vi "Append Line.vi"(0 "PDF Report IN":T22(xcontrol), 1 "Line cluster":T1={"Thickness (point)"=0.75, "Alighment"=enum."Right", "%width"=100.0, "Color"=1, "X Offset (point)"=0.0, "Y Offset (point)"=-6.0} {"%width" min=0 max=100 format="%#.0f"}, 11 "error in (no error)":errorcluster) -> (4 "PDF Report OUT":T22(xcontrol), 15 "error out":errorcluster)   [LabVIEW 2013]
doc: "<B>ENGLISH</B>\nAppends a <B>horizontal line</B> to the PDF report.\n\n<B>FRANÇAIS</B>\nAjoute une <B>ligne horizontale</B> au rapport PDF.\n\nDeveloped by Jean-Marc Simard\nCopyright © 2010, Exaprom Inc.\nAll rights reserved.\nLicense: BSD\n\nWith iTextSharp 4.1.6 (http://itextsharp.sourceforge.net)\nunder Mozilla Public License Version 1.1\n(http://www.mozilla.org/MPL/MPL-1.1.html)"
uses:
  C:/Users/MaxCorp/Documents/GitHub/TopView/DLL/itextsharp.dll
  DLL/itextsharp.dll
  Controls/CB SetColor.ctl
  Controls/Line cluster.ctl
  Controls/PDF Report Xcontrol/PDF Report.xctl
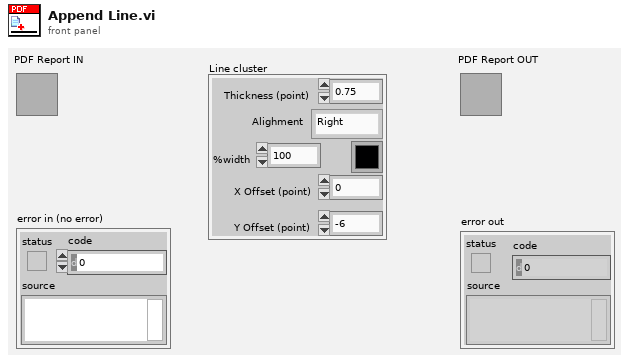
[diagram p1: front panel]
types:
  T1 = typedef "Line cluster.ctl" = cluster{"Thickness (point)":sgl, "Alighment":enum16{"Left", "Center", "Right"}, "%width":sgl, "Color":u32, "X Offset (point)":sgl, "Y Offset (point)":sgl}
  T2 = typedef "Font cluster.ctl" = cluster{"Name":string, "Size":T3, "Color":T4, "Style":cluster{"Bold":bool, "Italic":bool, "Underline":bool, "Strikeout":bool}}
  T3 = typedef "Font size.ctl" = sgl
  T4 = typedef "Font color.ctl" = u32
  T5 = typedef "Unit.ctl" = enum16{"inch", "mm"}
  T6 = typedef "Paragraphe cluster.ctl" = cluster{" Aligment":T7, "Line spacing":T8}
  T7 = typedef "Texte alignement.ctl" = enum16{"Select", "CENTER", "JUSTIFY", "LEFT", "RIGHT"}
  T8 = typedef "Line spacing.ctl" = enum16{"Select", "1.0", "1.5", "2.0"}
  T9 = typedef "Page dimensions.ctl" = cluster{"Start at page":i32, "Orientation":T10, "widht":sgl, "height":sgl, "Margin left":sgl, "Margin right":sgl, "Margin top":sgl, "Margin bottom":sgl}
  T10 = typedef "Page Orientation.ctl" = enum16{"Portrait", "Landscape"}
  T11 = typedef "Image or Table Caption.ctl" = cluster{"Caption":string, "Separator":string, "Position":enum16{"Above", "Below"}}
  T12 = typedef "Header Footer [ ].ctl" = T13[]
  T13 = typedef "Header Footer cluster.ctl" = cluster{"Start page":i32, "Type":T14, "Alignment":T15, "Vertical Alignement":T16, "Image (%)":sgl, "Page #":T17, "Text":string, "Path":string, "Font":T2, "Font refnum":refnum<k24>, "Line":cluster{"Line":T18, "Thickness (points)":sgl, "Colour":T4}}
  T14 = typedef "Header Footer Type.ctl" = enum16{"Select", "Text", "Text + hyperlink", "Page number", "Image", "Image + hyperlink"}
  T15 = typedef "Header footer horiz alignment.ctl" = enum16{"Left", "Center", "Right"}
  T16 = typedef "Cell Vertical alignment.ctl" = enum16{"TOP", "MIDDLE", "BOTTOM"}
  T17 = typedef "Page number.ctl" = cluster{"Text 1":string, "Text 2":string, "Text 3":string}
  T18 = typedef "Header Footer Line.ctl" = enum16{"No line", "Horizontal line"}
  T19 = typedef "Watermark cluster2.ctl" = cluster{"Show? (F)":bool, "Type":enum16{"Image", "Text"}, "Opacity (%)":sgl, "Rotate(°)":sgl, "Position":cluster{"Position":T20, "X":sgl, "Y":sgl}, "Image path":path, "Scaled(%)":sgl, "Image refnum":refnum<k24>, "Text":string, "Font":cluster{"Name":string, "Size":T3, "Color":T4}, "Font refnum":refnum<k24>, "Alignment":T15, "Automatic":bool}
  T20 = typedef "Watermark Position.ctl" = enum16{"Absolute", "Center (page)", "Center (text section)"}
  T21 = typedef "System Fonts.ctl" = cluster{"Font name [ ]":string[], "Font and file names [ ]":cluster{"Font name":string, "File name":string}[]}
  T22 = cluster{"Document":refnum<k24>, "Writer":refnum<k24>, "Default Font":refnum<k24>, "Default Font cluster":T2, "Path":path, "Unit (default = mm)":T5, "Paragraphe cluster":T6, "Pages dimensions [ ]":T9[], "Captions":cluster{"Image":T11, "Image counter":u16, "Table":T11, "Table counter":u16, "Font":T2}, "Header":T12, "Footer":T12, "Watermark ":T19, "Actual VI name":string, "System Fonts":T21}
  T23 = typedef "CB SetColor.ctl" = enum16{"Fill", "Stroke"}
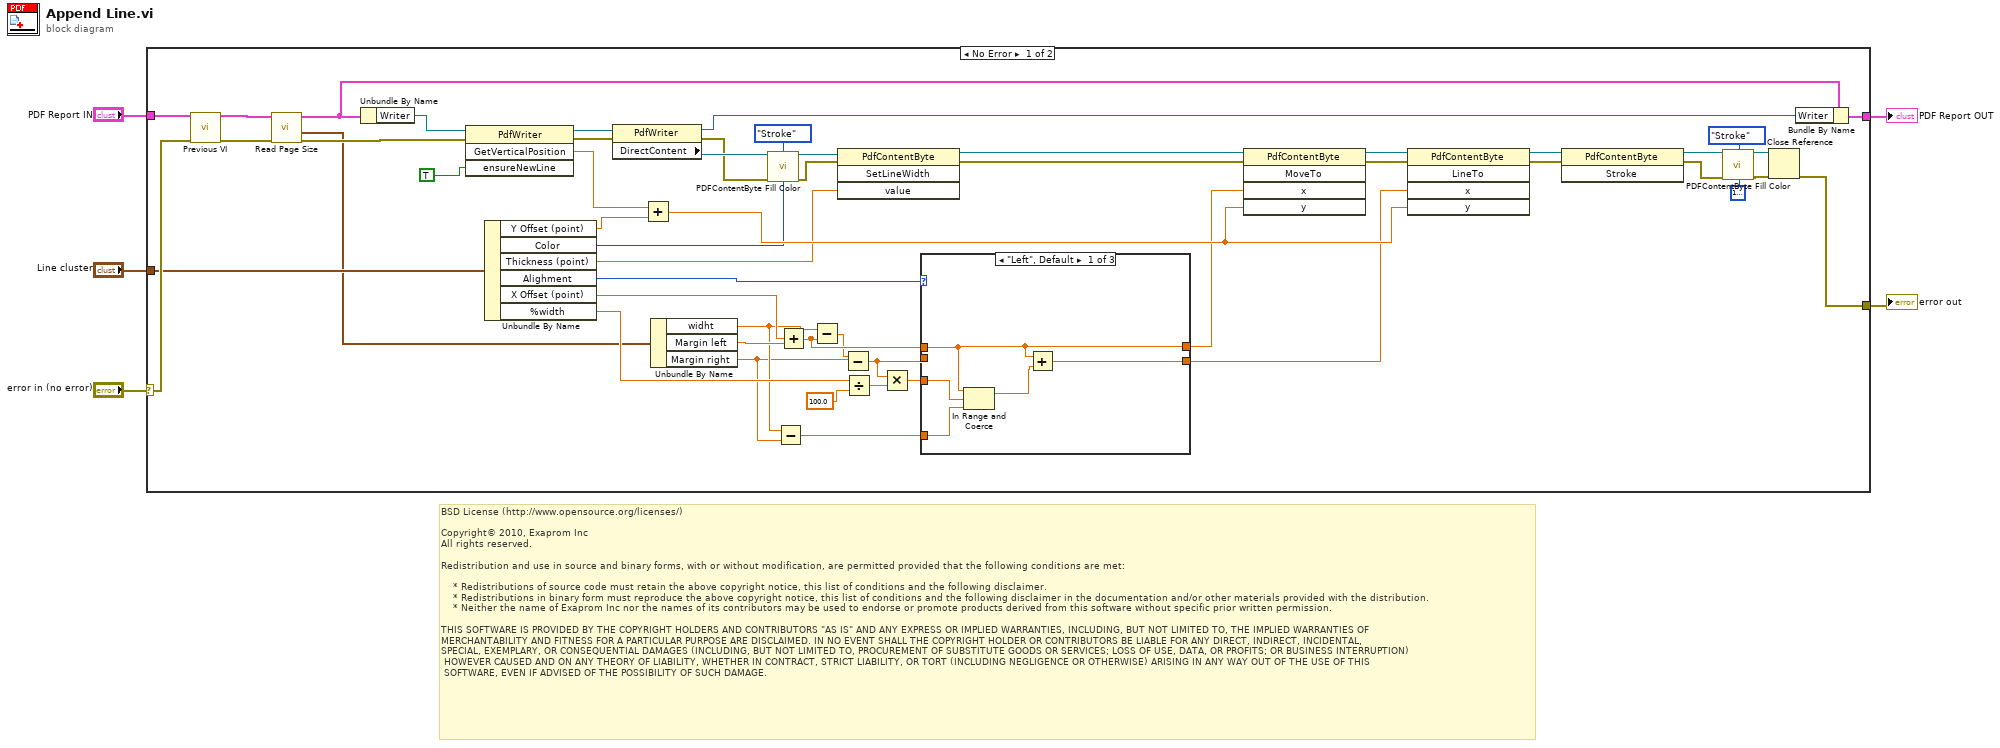
[diagram p0: block diagram]
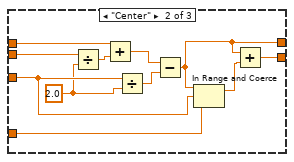
[diagram p2: hidden frame]
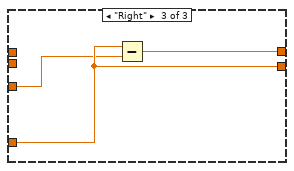
[diagram p3: hidden frame]
diagram:
  # "BSD License (http://www.opensource.org/licenses/)\n\nCopyright© 2010, Exaprom Inc\nAll rights reserved.\n\nRedistribution and use in source and binary forms, with or without modification, are permitted provided that the following conditions are met:\n\n    * Redistributions of source code must retain the above copyright notice, this list of conditions and the following disclaimer.\n    * Redistributions in binary form must reproduce the above copyright notice, this list of conditions and the following disclaimer in the documentation and/or other materials provided with the distribution.\n    * Neither the name of Exaprom Inc nor the names of its contributors may be used to endorse or promote products derived from this software without specific prior written permission.\n\nTHIS SOFTWARE IS PROVIDED BY THE COPYRIGHT HOLDERS AND CONTRIBUTORS \"AS IS\" AND ANY EXPRESS OR IMPLIED WARRANTIES, INCLUDING, BUT NOT LIMITED TO, THE IMPLIED WARRANTIES OF \nMERCHANTABILITY AND FITNESS FOR A PARTICULAR PURPOSE ARE DISCLAIMED. IN NO EVENT SHALL THE COPYRIGHT HOLDER OR CONTRIBUTORS BE LIABLE FOR ANY DIRECT, INDIRECT, INCIDENTAL,\nSPECIAL, EXEMPLARY, OR CONSEQUENTIAL DAMAGES (INCLUDING, BUT NOT LIMITED TO, PROCUREMENT OF SUBSTITUTE GOODS OR SERVICES; LOSS OF USE, DATA, OR PROFITS; OR BUSINESS INTERRUPTION)\n HOWEVER CAUSED AND ON ANY THEORY OF LIABILITY, WHETHER IN CONTRACT, STRICT LIABILITY, OR TORT (INCLUDING NEGLIGENCE OR OTHERWISE) ARISING IN ANY WAY OUT OF THE USE OF THIS\n SOFTWARE, EVEN IF ADVISED OF THE POSSIBILITY OF SUCH DAMAGE."
  n1 = case shown="No Error" "error in (no error)" {
    selector: "error in (no error)" -> [w57 w78]
    tunnel: [w20 w78] -> w5
    tunnel: "PDF Report IN" -> [w24 w77]
    tunnel: [w27 w77] -> w2
    tunnel: "Line cluster" -> [w42 _]
    frame No Error {
      n2 = call "Previous VI.vi"("PDF Report IN"=w24, "error in (no error)"=w57) -> ("PDF Report OUT"=w7:T22, "error out"=w6:errorcluster)  [unwired: 12 out]
      n3 = call "Read Page Size.vi"("error in (no error)"=w6, "PDF Report"=w7) -> ("error out"=w22:errorcluster, "Page (points)"=w21:T9, "PDF Report duplicate"=w23:T22)  [unwired: 7 out]
      n4 = Unbundle By Name(w23) -> ("Writer"=w26:refnum<k24>)
      n5 = invoke class="PdfWriter" method="GetVerticalPosition"(reference=w26, error in=w22, "ensureNewLine"=TRUE) -> (reference out=w55:refnum<k24>, error out=w56:errorcluster, "GetVerticalPosition"=w49:sgl)  [unwired: 1 in, 1 out]
      n6 = Unbundle By Name(w42) -> ("Y Offset (point)"=w41:sgl, "Color"=w10:u32, "Thickness (point)"=w40:sgl, "Alighment"=w38:enum16{"Left", "Center", "Right"}, "X Offset (point)"=w36:sgl, "%width"=w39:sgl)
      n7 = property class="PdfWriter"(reference=w55, error in=w56) -> (reference out=w25:refnum<k24>, error out=w12:errorcluster, "DirectContent"=w13:refnum<k24>)
      n8 = Add(x=w49, y=w41) -> (x+y=w48:sgl)
      n9 = Unbundle By Name(w21) -> ("widht"=w34:sgl, "Margin left"=w37:sgl, "Margin right"=w32:sgl)
      n10 = call "PDFContentByte Fill Color.vi"("PDFContentByte"=w13, "CB SetColor"=CB_SetColor."Stroke", "error in (no error)"=w12, "Color Box"=w10) -> ("PDFContentByte duplicate"=w14:refnum<k24>, "error out"=w11:errorcluster)  [unwired: 10 out]
      n11 = Subtract(x=w34, y=w32) -> (x-y=w33:sgl)
      n12 = Add(x=w36, y=w37) -> (x+y=w35:sgl)
      n13 = Subtract(x=w34, y=w35) -> (x-y=w31:sgl)
      n14 = invoke class="PdfContentByte" method="SetLineWidth"(reference=w14, error in=w11, "value"=w40) -> (reference out=w29:refnum<k24>, error out=w28:errorcluster)  [unwired: 1 in, 2 out]
      n15 = Subtract(x=w31, y=w32) -> (x-y=w30:sgl)
      n16 = Divide(x=w39, y=sgl 100.0) -> (x/y=w43:sgl)
      n17 = Multiply(x=w30, y=w43) -> (x*y=w46:sgl)
      n18 = case shown="\"Left\", Default" w38 {
        tunnel: w35 -> [w60 w69 _]
        tunnel: [w60 w66 w75] -> w47
        tunnel: w46 -> [w59 w65 w74]
        tunnel: [w62 w73 w76] -> w45
        tunnel: w33 -> [w61 w64 w76]
        tunnel: w30 -> [_ w71 _]
        frame "Left", Default {
          n19 = In Range and Coerce(upper limit=w60, x=w59, lower limit=w61) -> (coerced(x)=w58:sgl)  [unwired: 1 out]
          n20 = Add(x=w60, y=w58) -> (x+y=w62:sgl)
        }
        frame "Center" {
          w63 = sgl 2.0 ("y")
          n21 = Divide(x=w71, y=w63) -> (x/y=w70:sgl)
          n22 = Add(x=w69, y=w70) -> (x+y=w67:sgl)
          n23 = Divide(x=w65, y=w63) -> (x/y=w68:sgl)
          n24 = Subtract(x=w67, y=w68) -> (x-y=w66:sgl)
          n25 = In Range and Coerce(upper limit=w66, x=w65, lower limit=w64) -> (coerced(x)=w72:sgl)  [unwired: 1 out]
          n26 = Add(x=w66, y=w72) -> (x+y=w73:sgl)
        }
        frame "Right" {
          n27 = Subtract(x=w76, y=w74) -> (x-y=w75:sgl)
        }
      }
      n28 = invoke class="PdfContentByte" method="MoveTo"(reference=w29, error in=w28, "x"=w47, "y"=w48) -> (reference out=w50:refnum<k24>, error out=w53:errorcluster)  [unwired: 1 in, 3 out]
      n29 = invoke class="PdfContentByte" method="LineTo"(reference=w50, error in=w53, "x"=w45, "y"=w48) -> (reference out=w51:refnum<k24>, error out=w52:errorcluster)  [unwired: 1 in, 3 out]
      n30 = invoke class="PdfContentByte" method="Stroke"(reference=w51, error in=w52) -> (reference out=w18:refnum<k24>, error out=w19:errorcluster)  [unwired: 1 in, 1 out]
      n31 = call "PDFContentByte Fill Color.vi"("PDFContentByte"=w18, "CB SetColor"=CB_SetColor."Stroke", "error in (no error)"=w19, "Color Box"=u32 16777222) -> ("PDFContentByte duplicate"=w17:refnum<k24>, "error out"=w16:errorcluster)  [unwired: 10 out]
      n32 = Close Reference(reference=w17, error in (no error)=w16) -> (error out=w20:errorcluster)
      n33 = Bundle By Name(cluster=w23, "Writer"=w25) -> (w27:T22)
    }
    frame Error {
    }
  }
  "error out" <- w5
  "PDF Report OUT" <- w2
